vi "Example.vi"() -> ()   [LabVIEW 2018, in "QueueTimer.lvlib"]
doc: "Open and run the `Example.vi` to see how to use this queue timer library.\n\nRefer to the block diagram labels for more information."
uses:
  QueueTimer.lvlib
panel:
  in  "Start All":bool
  in  "Stop All":bool
  in  "msg1 Start":bool
  in  "msg1 Stop":bool
  out "Last Ticks (ms)":u32[](array[numeric])
  out "Running":bool[](array[boolean])
  out "Delay (ms)":i32[](array[numeric])
  out "Timer Messages":string[](array[string])
  in  "Stop":bool
  out "ms Destroy":u32
  out "msg2 time":timestamp format="%<%Y-%m-%d %H:%M:%S%6u>T"
  out "msg1 time":timestamp format="%<%Y-%m-%d %H:%M:%S%6u>T"
  out "msg1 count":i32
  out "msg2 count":i32
  out "Error":errorcluster
  # "Timer 1: \"msg1\""
  # "Timer 2: \"msg2\""
  # "Status"
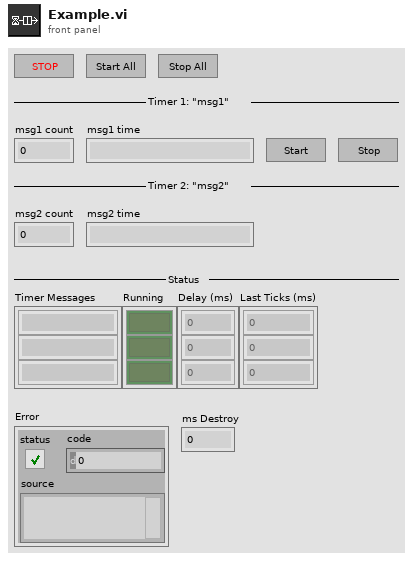
[diagram p1: front panel]
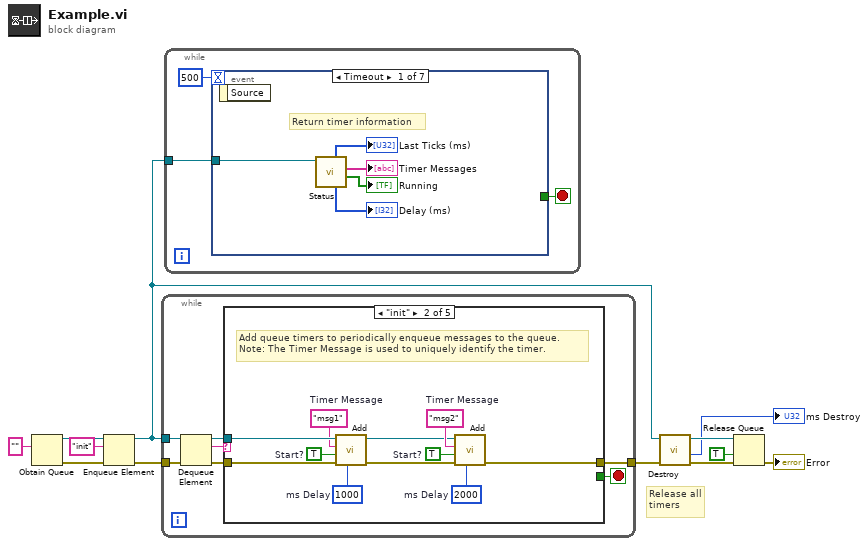
[diagram p0: block diagram]
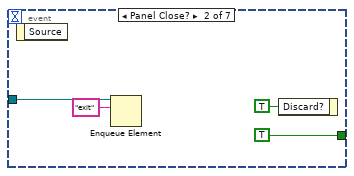
[diagram p2: hidden frame]
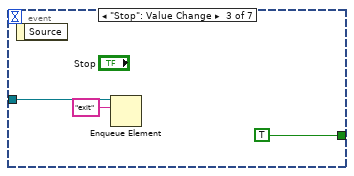
[diagram p3: hidden frame]
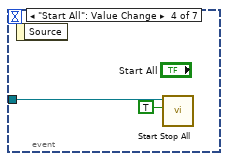
[diagram p4: hidden frame]
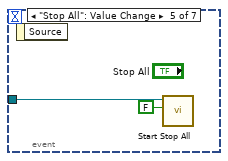
[diagram p5: hidden frame]
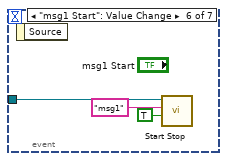
[diagram p6: hidden frame]
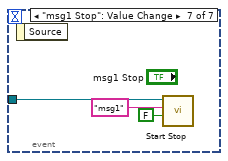
[diagram p7: hidden frame]
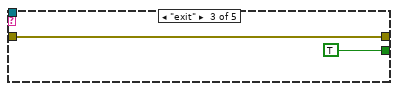
[diagram p9: hidden frame]
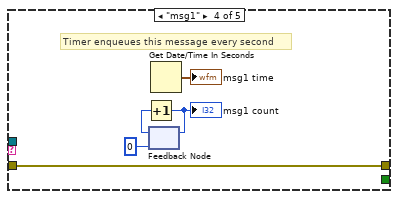
[diagram p10: hidden frame]
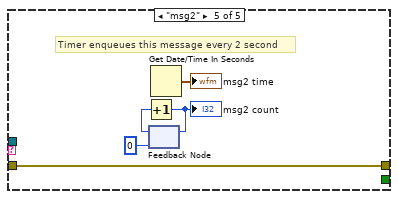
[diagram p11: hidden frame]
diagram:
  # "Release all\ntimers"
  n1 = Obtain Queue(element data type="") -> (queue out=w4:refnum<queue>, error out=w5:errorcluster)  [unwired: 4 in, 1 out]
  n2 = Enqueue Element(queue=w4, element="init", error in (no error)=w5) -> (queue out=w10:refnum<queue>, error out=w12:errorcluster)  [unwired: 1 in, 1 out]
  n3 = while {
    tunnel: w12 -> [w19]
    tunnel: w10 -> [w18]
    tunnel: [w16] -> w8
    stop <- w13 stop-if-true
    n4 = Dequeue Element(queue=w18, error in (no error)=w19) -> (queue out=w14:refnum<queue>, element=w17:string, error out=w15:errorcluster)  [unwired: 1 in, 1 out]
    n5 = case shown="\"init\"" w17 {
      tunnel: [w20 w27 w32 w38 w43] -> w16
      tunnel: w15 -> [w20 w31 w32 w38 w43]
      tunnel: w14 -> [_ w30 _ _ _]
      tunnel: [_ _ TRUE _ _] -> w13
      frame Default {
      }
      frame "init" {
        w22 = TRUE  # Start?
        w24 = TRUE  # Start?
        w21 = 2000  # ms Delay
        w28 = "msg2"  # Timer Message
        w23 = 1000  # ms Delay
        w29 = "msg1"  # Timer Message
        # "Add queue timers to periodically enqueue messages to the queue.\nNote: The Timer Message is used to uniquely identify the timer."
        n6 = call "Add.vi"("ms Delay (1000)"=w23, "error in (no error)"=w31, "Start? (T)"=w24, "Timer Message"=w29, "Queue in"=w30) -> ("error out"=w25:errorcluster, "Queue out"=w26:refnum<queue>)  [unwired: 4 in, 1 out]
        n7 = call "Add.vi"("ms Delay (1000)"=w21, "error in (no error)"=w25, "Start? (T)"=w22, "Timer Message"=w28, "Queue in"=w26) -> ("error out"=w27:errorcluster)  [unwired: 4 in, 2 out]
      }
      frame "exit" {
      }
      frame "msg1" {
        # "Timer enqueues this message every second"
        n8 = feedback #1(0) -> (w37:i32)
        n9 = Increment(x=w37) -> (x+1=w36:i32)
        "msg1 count" <- w36
        n10 = feedback-in #1(w36) -> ()
        n11 = Get Date/Time In Seconds() -> (seconds since 1Jan1904=→"msg1 time":timestamp)
      }
      frame "msg2" {
        # "Timer enqueues this message every 2 second"
        n12 = feedback #2(0) -> (w41:i32)
        n13 = Increment(x=w41) -> (x+1=w40:i32)
        "msg2 count" <- w40
        n14 = feedback-in #2(w40) -> ()
        n15 = Get Date/Time In Seconds() -> (seconds since 1Jan1904=→"msg2 time":timestamp)
      }
    }
  }
  n16 = while {
    tunnel: w10 -> [w45]
    stop <- w46 stop-if-true
    n17 = event shown="[0] Timeout" {
      selector: _ -> [_ _ _ _ _ _ _]
      dyn-events: _ -> [_ _ _ _ _ _ _]
      timeout: 500 -> [_ _ _ _ _ _ _]
      tunnel: [_ TRUE ("Discard?") TRUE ("Discard?") _ _ _ _] -> w46
      tunnel: w45 -> [w51 w53 w57 w60 w62 w65 w68]
      event Timeout {
        # "Return timer information"
        n18 = event-data() -> ()  [unwired: 1 in, 1 out]
        n19 = call "Status.vi"("Queue in"=w51) -> ("Running"=→"Running":bool[], "Timer Messages"=→"Timer Messages":string[], "Delay (ms)"=→"Delay (ms)":i32[], "Last Ticks (ms)"=→"Last Ticks (ms)":u32[])  [unwired: 5 in, 2 out]
      }
      event Panel Close? {
        n20 = event-data() -> ()  [unwired: 1 in, 1 out]
        n21 = Enqueue Element(queue=w53, element="exit" ("Message")) -> ()  [unwired: 2 in, 3 out]
        n22 = event-data("Discard?"=TRUE) -> ()  [unwired: 1 in, 1 out]
      }
      event "Stop": Value Change {
        n23 = event-data() -> ()  [unwired: 1 in, 1 out]
        n24 = Enqueue Element(queue=w57, element="exit" ("Message")) -> ()  [unwired: 2 in, 3 out]
      }
      event "Start All": Value Change {
        n25 = event-data() -> ()  [unwired: 1 in, 1 out]
        n26 = call "Start Stop All.vi"("Start? (T)"=TRUE, "Queue in"=w60) -> ()  [unwired: 7 in, 3 out]
      }
      event "Stop All": Value Change {
        n27 = event-data() -> ()  [unwired: 1 in, 1 out]
        n28 = call "Start Stop All.vi"("Start? (T)"=FALSE, "Queue in"=w62) -> ()  [unwired: 7 in, 3 out]
      }
      event "msg1 Start": Value Change {
        n29 = event-data() -> ()  [unwired: 1 in, 1 out]
        n30 = call "Start Stop.vi"("Start? (T)"=TRUE, "Timer Message"="msg1", "Queue in"=w65) -> ()  [unwired: 7 in, 2 out]
      }
      event "msg1 Stop": Value Change {
        n31 = event-data() -> ()  [unwired: 1 in, 1 out]
        n32 = call "Start Stop.vi"("Start? (T)"=FALSE, "Timer Message"="msg1", "Queue in"=w68) -> ()  [unwired: 7 in, 2 out]
      }
    }
  }
  n33 = call "Destroy.vi"("error in (no error)"=w8, "Queue in"=w10) -> ("error out"=w7:errorcluster, "ms Elapsed"=→"ms Destroy":u32, "Queue out"=w9:refnum<queue>)  [unwired: 7 in]
  n34 = Release Queue(queue=w9, force destroy? (F)=TRUE, error in (no error)=w7) -> (error out=→"Error":errorcluster)  [unwired: 2 out]
